vi "kADPosMerge2.vi"(8 "Mismatch Tol":dbl=0.1, 9 "EncoderCountTimed":i32, 10 "B Analog Encoder Sync":i16, 11 "A Analog Encoder Sync":i16) -> (1 "AD Mismatch":u16, 3 "Final Position":dbl)   [LabVIEW 2010, in "KevLib01.lvlib"]
uses:
  KevLib01.lvlib
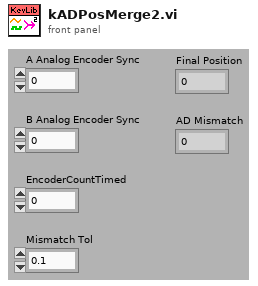
[diagram p1: front panel]
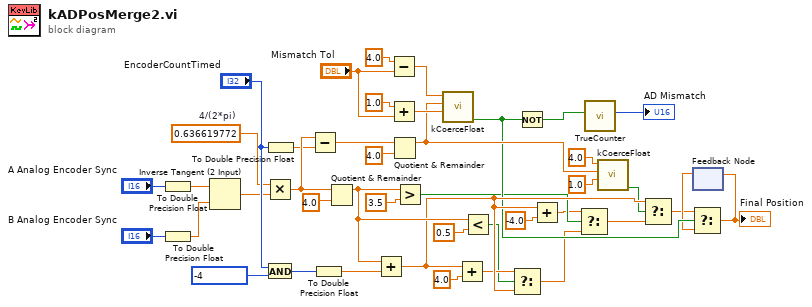
[diagram p0: block diagram]
diagram:
  w34 = 0.636619772  # 4/(2*pi)
  n1 = To Double Precision Float(number="A Analog Encoder Sync") -> (double precision float=w23:dbl)
  n2 = To Double Precision Float(number="B Analog Encoder Sync") -> (double precision float=w24:dbl)
  n3 = Inverse Tangent (2 Input)(1:w24, 2:w23) -> (0:w33:dbl)
  n4 = Multiply(x=w34, y=w33) -> (x*y=w36:dbl)
  n5 = And(x="EncoderCountTimed", y=-4) -> (x .and. y?=w38:i32)
  n6 = To Double Precision Float(number="EncoderCountTimed") -> (double precision float=w32:dbl)
  n7 = Subtract(x=w36, y=w32) -> (x-y=w27:dbl)
  n8 = To Double Precision Float(number=w38) -> (double precision float=w39:dbl)
  n9 = Quotient & Remainder(x=w36, y=4.0) -> (x-y*floor(x/y)=w42:dbl)  [unwired: 1 out]
  n10 = Add(x=w42, y=w39) -> (x+y=w41:dbl)
  n11 = Subtract(x=4.0 ("y"), y="Mismatch Tol") -> (x-y=w21:dbl)
  n12 = Add(x=1.0 ("y"), y="Mismatch Tol") -> (x+y=w20:dbl)
  n13 = Quotient & Remainder(x=w27, y=4.0) -> (x-y*floor(x/y)=w19:dbl)  [unwired: 1 out]
  n14 = Greater?(x=w42, y=3.5) -> (0:w10:bool)
  n15 = call "kCoerceFloat.vi"("lower"=w20, "input"=w19, "upper"=w21) -> ("coerced?"=w17:bool)  [unwired: 8 out]
  n16 = Add(x=w41, y=4.0) -> (x+y=w5:dbl)
  n17 = Less?(x=w42, y=0.5) -> (x < y?=w4:bool)
  n18 = Select(t=w5, s=w4, f=w41) -> (s? t:f=w8:dbl)
  n19 = Not(x=w17) -> (.not. x?=w18:bool)
  n20 = Add(x=w41, y=-4.0) -> (x+y=w9:dbl)
  n21 = Select(t=w9, s=w10, f=w8) -> (s? t:f=w3:dbl)
  n22 = call "TrueCounter.vi"("True?"=w18) -> ("True Count"=→"AD Mismatch":u16)  [unwired: 10 out]
  n23 = call "kCoerceFloat.vi"("lower"=1.0 ("y"), "input"=w19, "upper"=4.0 ("y")) -> ("coerced?"=w13:bool)  [unwired: 8 out]
  n24 = Select(t=w41, s=w13, f=w3) -> (s? t:f=w2:dbl)
  n25 = feedback #1() -> (w16:dbl)  [unwired: 1 out]
  n26 = Select(t=w2, s=w17, f=w16) -> (s? t:f=w1:dbl)
  "Final Position" <- w1
  n27 = feedback-in #1(w1) -> ()
